vi "write-hdf5-attributes.vi"(8 "error in (no error)":errorcluster, 11 "dset ref in":T1 format="%.0x") -> (0 "error out":errorcluster, 3 "dset ref out":T1 format="%.0x")   [LabVIEW 2016]
uses:
  <vilib>/addons/h5labview2/base/hid_t.ctl
  <vilib>/addons/h5labview2/base/lib_path.vi
  <vilib>/addons/h5labview2/base/H5Equery.vi
  <vilib>/addons/h5labview2/attrib/H5Awrite.llb/H5Awrite.xnode
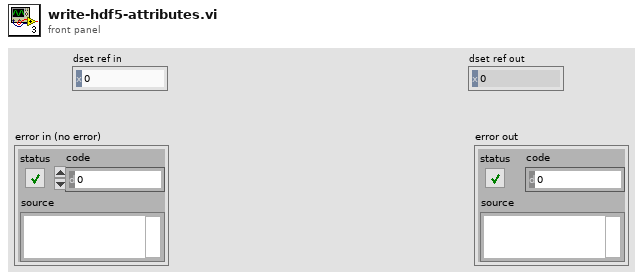
[diagram p1: front panel]
types:
  T1 = typedef "hid_t.ctl" = i32
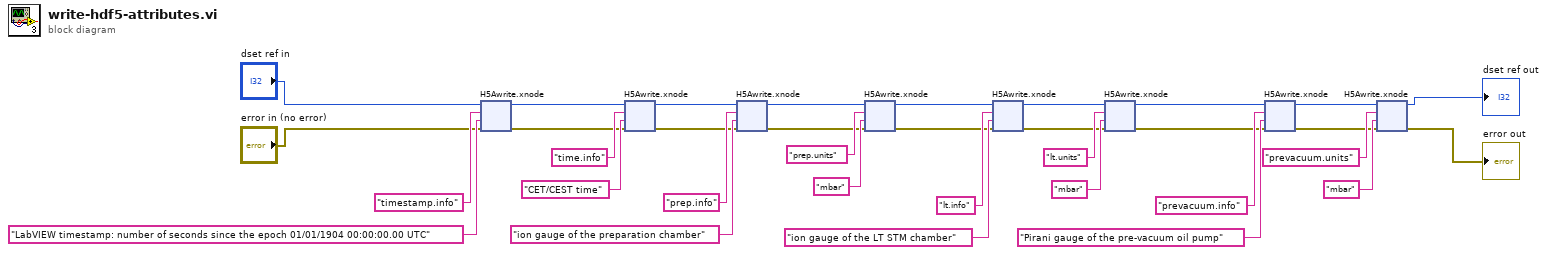
[diagram p0: block diagram]
diagram:
  n1 = xnode "H5Awrite.xnode"("error in (no error)"="error in (no error)", "data"="LabVIEW timestamp: number of seconds since the epoch 01/01/1904 00:00:00.00 UTC" ("attrib name"), "attrib name"="timestamp.info", "ref in"="dset ref in") -> ("error out"=w3:errorcluster, "ref out"=w6:i32)  [unwired: 3 in, 1 out]
  n2 = xnode "H5Awrite.xnode"("error in (no error)"=w3, "data"="CET/CEST time" ("attrib name"), "attrib name"="time.info", "ref in"=w6) -> ("error out"=w4:errorcluster, "ref out"=w5:i32)  [unwired: 3 in, 1 out]
  n3 = xnode "H5Awrite.xnode"("error in (no error)"=w4, "data"="ion gauge of the preparation chamber" ("attrib name"), "attrib name"="prep.info", "ref in"=w5) -> ("error out"=w29:errorcluster, "ref out"=w30:i32)  [unwired: 3 in, 1 out]
  n4 = xnode "H5Awrite.xnode"("error in (no error)"=w29, "data"="mbar" ("attrib name"), "attrib name"="prep.units", "ref in"=w30) -> ("error out"=w15:errorcluster, "ref out"=w17:i32)  [unwired: 3 in, 1 out]
  n5 = xnode "H5Awrite.xnode"("error in (no error)"=w15, "data"="ion gauge of the LT STM chamber" ("attrib name"), "attrib name"="lt.info", "ref in"=w17) -> ("error out"=w14:errorcluster, "ref out"=w16:i32)  [unwired: 3 in, 1 out]
  n6 = xnode "H5Awrite.xnode"("error in (no error)"=w14, "data"="mbar" ("attrib name"), "attrib name"="lt.units", "ref in"=w16) -> ("error out"=w12:errorcluster, "ref out"=w13:i32)  [unwired: 3 in, 1 out]
  n7 = xnode "H5Awrite.xnode"("error in (no error)"=w12, "data"="Pirani gauge of the pre-vacuum oil pump" ("attrib name"), "attrib name"="prevacuum.info", "ref in"=w13) -> ("error out"=w10:errorcluster, "ref out"=w11:i32)  [unwired: 3 in, 1 out]
  n8 = xnode "H5Awrite.xnode"("error in (no error)"=w10, "data"="mbar" ("attrib name"), "attrib name"="prevacuum.units", "ref in"=w11) -> ("error out"=→"error out":errorcluster, "ref out"=→"dset ref out":i32)  [unwired: 3 in, 1 out]
